vi "formatOutputData.vi"(8 "error in (no error)":errorcluster, 10 "outputData":T1 {"Step & Direction" min=-32767}, 11 "Model in":refnum<class "Model.lvclass">) -> (0 "error out":errorcluster, 2 "outputDataString":string, 3 "Model out":refnum<class "Model.lvclass">)   [LabVIEW 2013, in "Model.lvclass"]
uses:
  Model.lvclass
  <userlib>/Common/ILC/Typedefs/OutputData.ctl
  <userlib>/Common/ILC/Typedefs/ILCTypedefs.lvlib
panel:
  # "DAC"
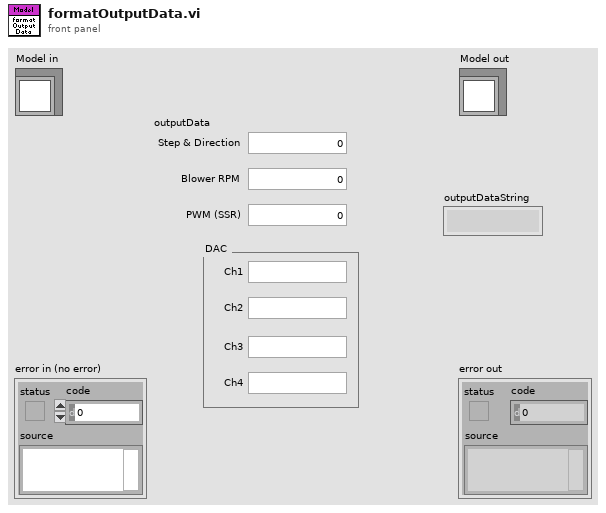
[diagram p1: front panel]
types:
  T1 = typedef "ILCCommon.lvlib/ILCTypedefs.lvlib/OutputData.ctl" = cluster{"Step & Direction":i16, "Blower RPM":u8, "PWM (SSR)":u8, "Ch1":u16, "Ch2":u16, "Ch3":u16, "Ch4":u16}
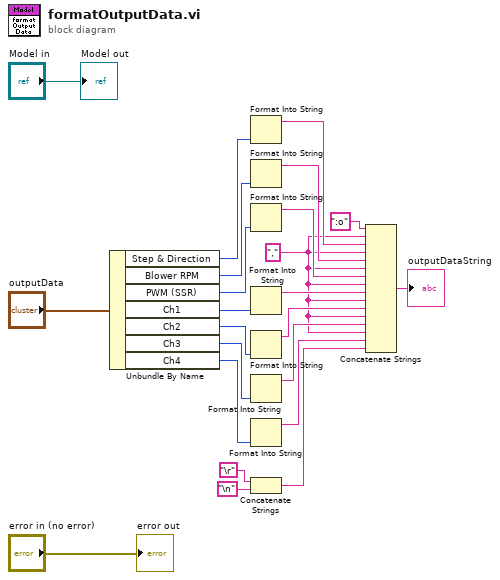
[diagram p0: block diagram]
diagram:
  w2 = "," ("string")
  n1 = Unbundle By Name("outputData") -> ("Step & Direction"=w19:i16, "Blower RPM"=w17:u8, "PWM (SSR)"=w15:u8, "Ch1"=w6:u16, "Ch2"=w5:u16, "Ch3"=w4:u16, "Ch4"=w3:u16)
  n2 = Format Into String(w19) -> (resulting string=w18:string)  [unwired: 3 in, 1 out]
  n3 = Format Into String(w17) -> (resulting string=w16:string)  [unwired: 3 in, 1 out]
  n4 = Format Into String(w15) -> (resulting string=w14:string)  [unwired: 3 in, 1 out]
  n5 = Format Into String(w6) -> (resulting string=w13:string)  [unwired: 3 in, 1 out]
  n6 = Format Into String(w5) -> (resulting string=w12:string)  [unwired: 3 in, 1 out]
  n7 = Format Into String(w4) -> (resulting string=w11:string)  [unwired: 3 in, 1 out]
  n8 = Format Into String(w3) -> (resulting string=w1:string)  [unwired: 3 in, 1 out]
  n9 = Concatenate Strings("\r", "\n") -> (w8:string)
  n10 = Concatenate Strings(":o" ("string"), w2, w18, w2, w16, w2, w14, w2, w13, w2, w12, w2, w11, w2, w1, w8) -> (→"outputDataString":string)
  "error out" <- "error in (no error)"
  "Model out" <- "Model in"
